vi "ex_4_10.vi"() -> ()   [LabVIEW 2020]
panel:
  out "Match Array":string[](array[string])
  in  "Match":string
  in  "String":string
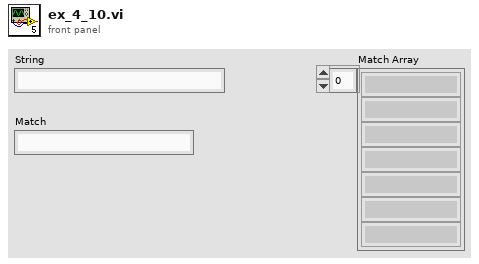
[diagram p1: front panel]
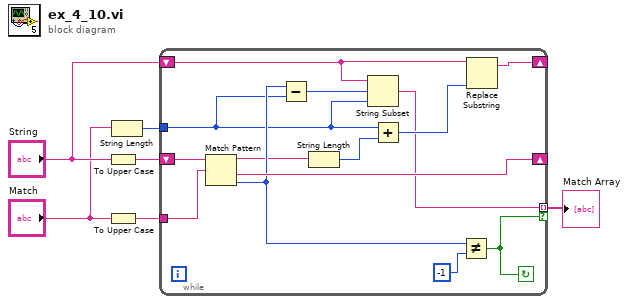
[diagram p0: block diagram]
diagram:
  n1 = To Upper Case(1:"String") -> (0:w6:string)
  n2 = To Upper Case(1:"Match") -> (0:w5:string)
  n3 = String Length(string="Match") -> (length=w3:i32)
  n4 = while {
    shift-right: [w18] -> _
    shift-left: w6 -> [w20]
    tunnel: w5 -> [w17]
    tunnel: [w8] -> w1 mode=indexing if=w16
    tunnel: w3 -> [w12]
    shift-right: [w9] -> _
    shift-left: "String" -> [w7]
    stop <- w16 continue-if-true
    n5 = Match Pattern(string=w20, regular expression=w17) -> (before substring=w13:string, after substring=w18:string, offset past match=w15:i32)  [unwired: 1 in, 1 out]
    n6 = Subtract(x=w15, y=w12) -> (x-y=w14:i32)
    n7 = String Length(string=w13) -> (length=w11:i32)
    n8 = String Subset(string=w7, offset (0)=w14, length (rest)=w12) -> (substring=w8:string)
    n9 = Add(x=w12, y=w11) -> (x+y=w10:i32)
    n10 = Not Equal?(x=w15, y=-1) -> (x != y?=w16:bool)
    n11 = Replace Substring(2:w10, 5:w7) -> (1:w9:string)  [unwired: 2 in, 1 out]
  }
  "Match Array" <- w1
